vi "Shutdown.vi"(8 "error in (no error)":errorcluster, 11 "UDPlog Transceiver in":refnum<class "UDPlog Transceiver.lvclass">) -> (0 "error out":errorcluster, 3 "UDPlog Transceiver out":refnum<class "UDPlog Transceiver.lvclass">)   [LabVIEW 2023, in "UDPlog.lvlib" / "UDPlog Transceiver.lvclass"]
uses:
  UDPlog Transceiver.lvclass
  UDPlog Transceiver.lvclass/UDPlog Transceiver.ctl
  Typedefs/Transfer Parameters.ctl
  Typedefs/Trasfer Group Parameters.ctl
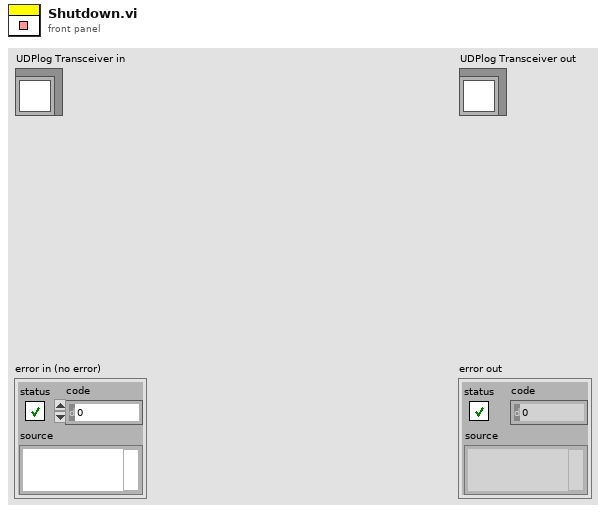
[diagram p1: front panel]
types:
  T1 = typedef "UDPlog.lvlib/UDPlog Transceiver.lvclass/Trasfer Group Parameters.ctl" = cluster{"transfers":T2[], "max size":i32, "timeout":i32}
  T2 = typedef "UDPlog.lvlib/UDPlog Transceiver.lvclass/Transfer Parameters.ctl" = cluster{"group offset":u64, "size":u64, "address":u32, "port":u16}
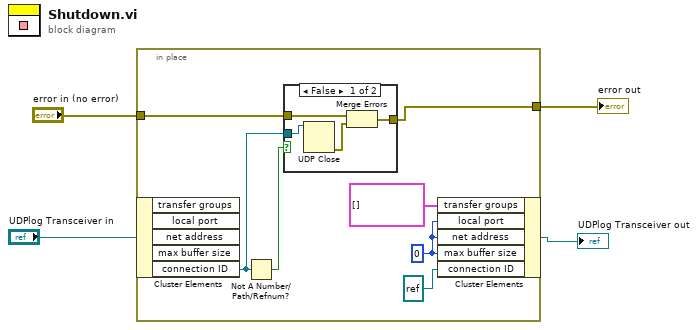
[diagram p0: block diagram]
diagram:
  n1 = in-place {
    in-place-border: "error in (no error)" -> [w9]
    in-place-border: [w5] -> w1
    w6 = u16 0 ("local port")
    n2 = in-place-cluster #1("UDPlog Transceiver in") -> ("connection ID"=w10:refnum<k16>)  [unwired: 4 out]
    n3 = Not A Number/Path/Refnum?(number/path/refnum=w10) -> (NaN/Path/Refnum?=w11:bool)
    n4 = case shown="False" w11 {
      tunnel: w9 -> [w14 w16]
      tunnel: [w13 w16] -> w5
      tunnel: w10 -> [w12 _]
      frame False {
        n5 = UDP Close(connection ID=w12) -> (error out=w15:errorcluster)  [unwired: 1 in, 1 out]
        n6 = Merge Errors(w14, w15) -> (w13:errorcluster)
      }
      frame True {
      }
    }
    n7 = in-place-cluster #1("transfer groups"=T1[] [], "local port"=w6, "net address"=w6, "max buffer size"=w6, "connection ID"=refnum<k16> refnum) -> (→"UDPlog Transceiver out":refnum<class "UDPlog Transceiver.lvclass">)
  }
  "error out" <- w1
